vi "Initialize from Config.vi"(8 "error in (no error)":errorcluster, 11 "Event Reporter Module in":refnum<class "Event Reporter Module.lvclass">) -> (0 "error out":errorcluster, 3 "Event Reporter Module out":refnum<class "Event Reporter Module.lvclass">)   [LabVIEW 2020, in "Volatus.lvlib" / "Event Reporter Module.lvclass"]
uses:
  Event Reporter Module.lvclass
  C:/dev/lv20CE/relink/lv-volatus/Volatus/Module/Module.lvclass
  VolatusConfig/Meta Type.ctl
  Module/Module.lvclass/Module.ctl
  VolatusConfig/VolatusConfigElement/VolatusConfigElement.lvclass/VolatusConfigElement.ctl
  Event Reporter Module.lvclass/Event Reporter Module.ctl
  Event.ctl
  Event Level.ctl
  VolatusConfig/VolatusConfigElement/Element.vi
  lv-cdm/CDM-Config/Config Lookup/Match Meta.vi
  lv-cdm/CDM-Config/Config Element/Owner.vi
  lv-cdm/CDM-Config/Config Filter/Config Lookup.lvclass
  Volatus.lvlib
  Module/Module.lvclass
  VolatusAPI/VolatusAPI.lvclass
  VolatusConfig/VolatusConfig.lvlib
  VolatusConfig/VolatusConfigElement/VolatusConfigElement.lvclass
  VolatusConfig/Node/Node.lvclass
  C:/dev/lv20CE/relink/lv-volatus/VolatusConfig/VolatusConfigElement/VolatusConfigElement.lvclass
  C:/dev/lv20CE/relink/lv-volatus/VolatusConfig/Node/Node.lvclass
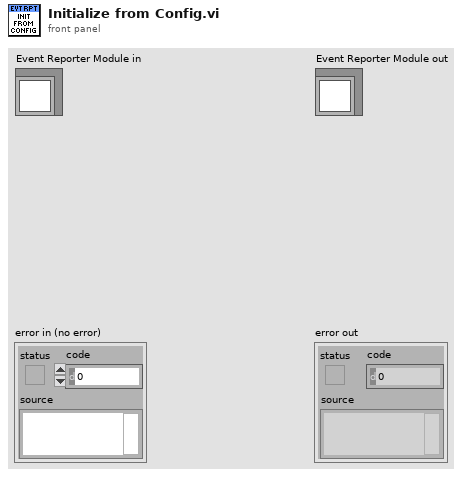
[diagram p1: front panel]
types:
  T1 = typedef "VolatusConfig.lvlib/Meta Type.ctl" = enum16{"UNKNOWN", "VL_System", "VL_Cluster", "VL_Node", "VL_Task", "VL_Group", "VL_Channel", "VL_Task_List", "VL_Scaling", "VL_Sensor", "VL_Sensor_List", "VL_Scale"}
  T2 = typedef "Volatus.lvlib/Event.ctl" = cluster{"Time Stamp":timestamp, "Event Level":T3, "Context":string, "Message":string, "Error":errorcluster, "Node":string}
  T3 = typedef "Volatus.lvlib/Event Level.ctl" = enum16{"Debug", "Info", "Warning", "Error"}
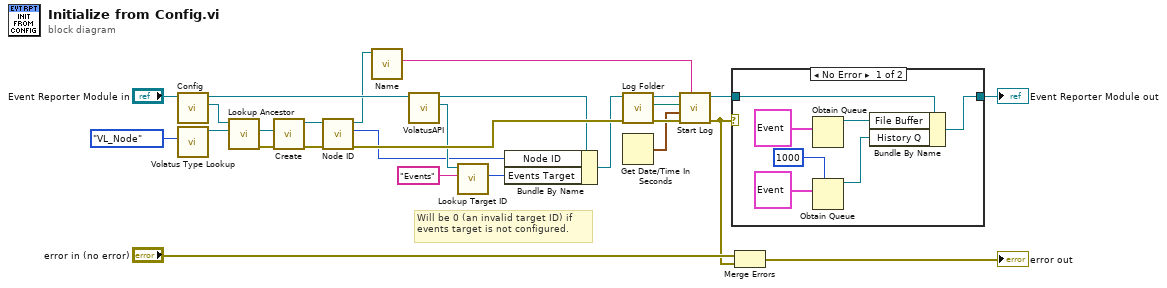
[diagram p0: block diagram]
diagram:
  # "Will be 0 (an invalid target ID) if events target is not configured."
  n1 = call "Config.vi"("Module in"="Event Reporter Module in") -> ("Config"=w9:refnum<class "VolatusConfigElement.lvclass">, "Module out"=w11:refnum<class "Event Reporter Module.lvclass">)  [unwired: 9 in]
  n2 = call "Volatus Type Lookup.vi"("Meta Type"=Meta_Type."VL_Node") -> ("Config Lookup out"=w8:refnum<class "Config Lookup.lvclass">)  [unwired: 9 in, 1 out]
  n3 = call "Lookup Ancestor.vi"("Lookup"=w8, "VolatusConfigElement in"=w9) -> ("error out"=w6:errorcluster, "Ancestor"=w7:refnum<class "Config Element.lvclass">)  [unwired: 7 in, 1 out]
  n4 = call "Create.vi"("error in (no error)"=w6, "Element"=w7) -> ("error out"=w4:errorcluster, "Node out"=w5:refnum<class "Node.lvclass">)  [unwired: 8 in]
  n5 = call "Node ID.vi"("error in (no error)"=w4, "Node in"=w5) -> ("error out"=w27:errorcluster, "Node ID"=w3:u32, "Node out"=w2:refnum<class "Node.lvclass">)  [unwired: 7 in]
  n6 = call "Name.vi"("VolatusConfigElement in"=w2) -> ("Name"=w1:string)  [unwired: 8 in, 2 out]
  n7 = call "VolatusAPI.vi"("Module in"=w11) -> ("VolatusAPI"=w16:refnum<class "VolatusAPI.lvclass">, "Module out"=w13:refnum<class "Event Reporter Module.lvclass">)  [unwired: 9 in]
  n8 = call "Lookup Target ID.vi"("Target Name"="Events", "VolatusAPI in"=w16) -> ("Target ID"=w14:u32)  [unwired: 7 in, 2 out]
  n9 = Bundle By Name(cluster=w13, "Node ID"=w3, "Events Target"=w14) -> (w12:refnum<class "Event Reporter Module.lvclass">)
  n10 = call "Log Folder.vi"("error in (no error)"=w27, "Event Reporter Module in"=w12) -> ("error out"=w26:errorcluster, "Log Folder"=w17:path, "Event Reporter Module out"=w18:refnum<class "Event Reporter Module.lvclass">)  [unwired: 7 in]
  n11 = Get Date/Time In Seconds() -> (seconds since 1Jan1904=w24:timestamp)
  n12 = call "Start Log.vi"("Node Name"=w1, "error in (no error)"=w26, "Time Stamp"=w24, "Folder"=w17, "Event Reporter Module in"=w18) -> ("error out"=w21:errorcluster, "Event Reporter Module out"=w22:refnum<class "Event Reporter Module.lvclass">)  [unwired: 5 in]
  n13 = case shown="No Error" w21 {
    tunnel: w22 -> [w32 w35]
    tunnel: [w31 w35] -> w20
    frame No Error {
      n14 = Obtain Queue(element data type=T2 {"Time Stamp"=timestamp(0 s since 1904-01-01), "Event Level"=enum."Info", "Context"="", "Message"="", "Error"={"status"=FALSE, "code"=0, "source"=""}, "Node"=""} ("Event")) -> (queue out=w33:refnum<queue>)  [unwired: 4 in, 2 out]
      n15 = Obtain Queue(max queue size (-1, unlimited)=1000, element data type=T2 {"Time Stamp"=timestamp(0 s since 1904-01-01), "Event Level"=enum."Info", "Context"="", "Message"="", "Error"={"status"=FALSE, "code"=0, "source"=""}, "Node"=""} ("Event")) -> (queue out=w28:refnum<queue>)  [unwired: 3 in, 2 out]
      n16 = Bundle By Name(cluster=w32, "File Buffer"=w33, "History Q"=w28) -> (w31:refnum<class "Event Reporter Module.lvclass">)
    }
    frame Error {
    }
  }
  "Event Reporter Module out" <- w20
  n17 = Merge Errors("error in (no error)", w21) -> (→"error out":errorcluster)
